vi "Match Type.vi"(7 "raise for mismatch?":bool, 8 "error in (no error)":errorcluster, 10 "type code":T1, 11 "NT Scalar in":refnum<class "NT Scalar.lvclass">) -> (0 "error out":errorcluster, 1 "type match?":bool, 2 "type code out":T1, 3 "NT Scalar out":refnum<class "NT Scalar.lvclass">)   [LabVIEW 2020, in "PV Access.lvlib" / "PV Data.lvlib" / "NT Scalar.lvclass"]
uses:
  NT Scalar.lvclass
  <vilib>/ErrorRing/Error Ring.xnode
  NT Scalar.lvclass/NT Scalar.ctl
  Type Code.ctl
  PV Data.lvlib
  <vilib>/Utility/error.llb/Error Cluster From Error Code.vi
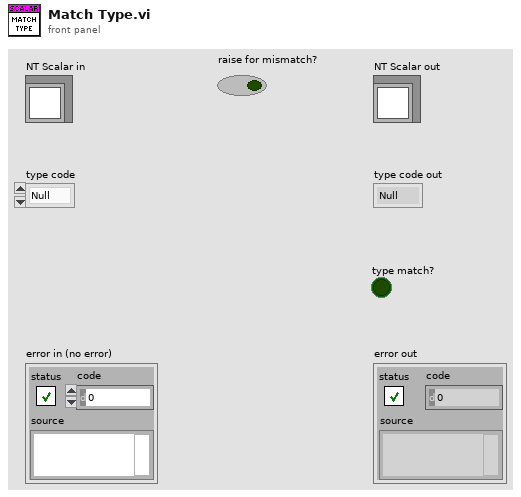
[diagram p1: front panel]
types:
  T1 = typedef "PV Access.lvlib/PV Data.lvlib/Type Code.ctl" = enum8{"Null", "Bool", "BoolA", "Int8", "Int8A", "Int16", "Int16A", "Int32", "Int32A", "Int64", "Int64A", "UInt8", "UInt8A", "UInt16", "UInt16A", "UInt32", "UInt32A", "UInt64", "UInt64A", "Float32", "Float32A", "Float64", "Float64A", "String", "StringA", "Struct", "StructA", "Union", "UnionA", "Any", "AnyA"}
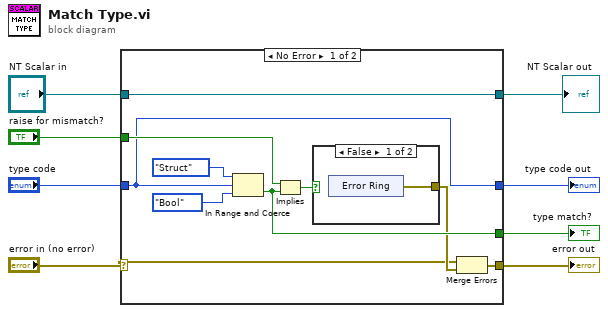
[diagram p0: block diagram]
diagram:
  n1 = case shown="No Error" "error in (no error)" {
    selector: "error in (no error)" -> [w11 w26]
    tunnel: [w10 w26] -> w4
    tunnel: [w18 w25] -> w2
    tunnel: "NT Scalar in" -> [w18 w25]
    tunnel: "type code" -> [w9 w24]
    tunnel: [w13 _] -> w3
    tunnel: "raise for mismatch?" -> [w15 _]
    tunnel: [w9 w24] -> w1
    frame No Error {
      n2 = In Range and Coerce(upper limit=Type_Code."Struct", x=w9, lower limit=Type_Code."Bool") -> (In Range?=w13:bool)  [unwired: 1 out]
      n3 = Implies(1:w13, 2:w15) -> (0:w14:bool)
      n4 = case shown="False" w14 {
        tunnel: [w19 _] -> w12
        frame False {
          n5 = xnode "Error Ring"() -> ("error out"=w19:errorcluster)
        }
        frame True {
        }
      }
      n6 = Merge Errors(w11, w12) -> (w10:errorcluster)
    }
    frame Error {
    }
  }
  "error out" <- w4
  "type match?" <- w3
  "NT Scalar out" <- w2
  "type code out" <- w1
